vi "Build FPGA Configuration.vi"(8 "error in (no error)":errorcluster, 11 "Item Ref in":T1 format="%.0x") -> (0 "error out":errorcluster, 2 "FPGA Configuration":refnum<k24>, 3 "Item Ref out":T1 format="%.0x")   [LabVIEW 2014, in "SLSC configuration System Explorer.lvlib"]
uses:
  SLSC configuration System Explorer.lvlib
  <vilib>/NI Veristand/Custom Device API/Custom Device Item Ref.ctl
  <vilib>/NI Veristand/Custom Device API/Custom Device API.lvlib
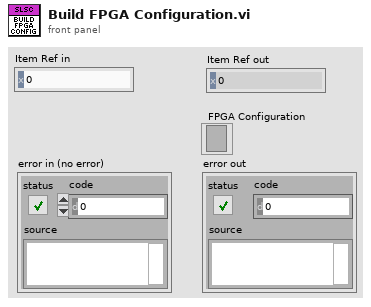
[diagram p1: front panel]
types:
  T1 = typedef "Custom Device API.lvlib/Custom Device Item Ref.ctl" = u64
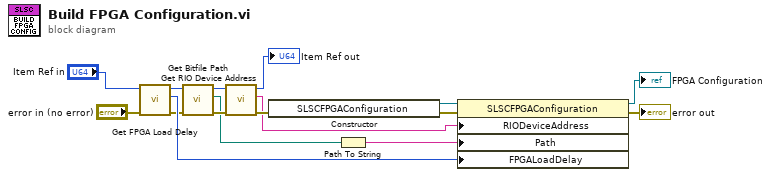
[diagram p0: block diagram]
diagram:
  n1 = call "Get FPGA Load Delay.vi"("error in (no error)"="error in (no error)", "Item Ref in"="Item Ref in") -> ("error out"=w6:errorcluster, "FPGA Load Delay (s)"=w14:u16, "Item Ref out"=w7:T1)  [unwired: 7 in]
  n2 = call "Get Bitfile Path.vi"("error in (no error)"=w6, "Item Ref in"=w7) -> ("error out"=w10:errorcluster, "Bitfile Path"=w8:path, "Item Ref out"=w11:T1)  [unwired: 7 in]
  n3 = call "Get RIO Device Address.vi"("error in (no error)"=w10, "Item Ref in"=w11) -> ("error out"=w13:errorcluster, "RIO Device Address"=w12:string, "Item Ref out"=→"Item Ref out":T1)  [unwired: 7 in]
  n4 = constructor class="SLSCFPGAConfiguration"(error in=w13) -> (reference out=w4:refnum<k24>, error out=w3:errorcluster)  [unwired: 2 in, 1 out]
  n5 = Path To String(path=w8) -> (string=w9:string)
  n6 = property class="SLSCFPGAConfiguration"(reference=w4, error in=w3, "RIODeviceAddress"=w12, "Path"=w9, "FPGALoadDelay"=w14) -> (reference out=→"FPGA Configuration":refnum<k24>, error out=→"error out":errorcluster)
